vi "UI_(02B)_Switch_to_offline_mode.vi"(6 "error in (no error)":errorcluster, 9 "Settings cluster in":T1={"Defaults"={"Default User"=0.0, "VISA Resource Name "="", "Histogram parameters"={"max"=300.0, "min"=0.0, "# bins"=10, "threshold"=8.0, "thr. type"=enum."higher accepted"}}, "Recording and saving"={"Researcher name"="", "Name prefix"="", "Data post-processing"={"Filter type"=enum."Savitzky-Golay", "Length"=31, "Order"=3}, "Stop at"=0.0, "\"Stop at\" enabled"=FALSE, "Default save folder path"=path "", "Acquisition FPS"=enum."Max"}, "Geometry"={"Sensor board size"=enum."", "Bridge swap"=FALSE, "Twisted neck"=FALSE, "Bridge H. offset"=0.0, "Bridge V. offset"=0.0, "Magnets orientation"=0.0, "Cage type"=0, "Cage parameters"={"Round"=variant(i16 0), "Square"=variant(u16 0), "Donut-maze"=variant(u16 0), "T-maze"=variant(u8 0), "Sociability-maze"=variant(u8 0)}}, "IO parameters"={"IO general config."=0, "IO 1 configuration"=0, "IO 2 configuration"=0, "IO 3 configuration"=0, "IO 4 configuration"=0, "Activate ext. RS-232"=0, "IO inversion config."=0, "Sync capability"=1}, "Conditions presets array"=[{"Enabled"=FALSE, "Name"="", "Specifier(s)"=[], "Response"={"Response type"=enum."Air puff", "TTL port"=enum."Port 1", "TTL pulse length, ms"=0.0}, "Has been set"=FALSE}, {"Enabled"=FALSE, "Name"="", "Specifier(s)"=[], "Response"={"Response type"=enum."Air puff", "TTL port"=enum."Port 1", "TTL pulse length, ms"=0.0}, "Has been set"=FALSE}, {"Enabled"=FALSE, "Name"="", "Specifier(s)"=[], "Response"={"Response type"=enum."Air puff", "TTL port"=enum."Port 1", "TTL pulse length, ms"=0.0}, "Has been set"=FALSE}, {"Enabled"=FALSE, "Name"="", "Specifier(s)"=[], "Response"={"Response type"=enum."Air puff", "TTL port"=enum."Port 1", "TTL pulse length, ms"=0.0}, "Has been set"=FALSE}, {"Enabled"=FALSE, "Name"="", "Specifier(s)"=[], "Response"={"Response type"=enum."Air puff", "TTL port"=enum."Port 1", "TTL pulse length, ms"=0.0}, "Has been set"=FALSE}, {"Enabled"=FALSE, "Name"="", "Specifier(s)"=[], "Response"={"Response type"=enum."Air puff", "TTL port"=enum."Port 1", "TTL pulse length, ms"=0.0}, "Has been set"=FALSE}, {"Enabled"=FALSE, "Name"="", "Specifier(s)"=[], "Response"={"Response type"=enum."Air puff", "TTL port"=enum."Port 1", "TTL pulse length, ms"=0.0}, "Has been set"=FALSE}, {"Enabled"=FALSE, "Name"="", "Specifier(s)"=[], "Response"={"Response type"=enum."Air puff", "TTL port"=enum."Port 1", "TTL pulse length, ms"=0.0}, "Has been set"=FALSE}, {"Enabled"=FALSE, "Name"="", "Specifier(s)"=[], "Response"={"Response type"=enum."Air puff", "TTL port"=enum."Port 1", "TTL pulse length, ms"=0.0}, "Has been set"=FALSE}, {"Enabled"=FALSE, "Name"="", "Specifier(s)"=[], "Response"={"Response type"=enum."Air puff", "TTL port"=enum."Port 1", "TTL pulse length, ms"=0.0}, "Has been set"=FALSE}, {"Enabled"=FALSE, "Name"="", "Specifier(s)"=[], "Response"={"Response type"=enum."Air puff", "TTL port"=enum."Port 1", "TTL pulse length, ms"=0.0}, "Has been set"=FALSE}, {"Enabled"=FALSE, "Name"="", "Specifier(s)"=[], "Response"={"Response type"=enum."Air puff", "TTL port"=enum."Port 1", "TTL pulse length, ms"=0.0}, "Has been set"=FALSE}, {"Enabled"=FALSE, "Name"="", "Specifier(s)"=[], "Response"={"Response type"=enum."Air puff", "TTL port"=enum."Port 1", "TTL pulse length, ms"=0.0}, "Has been set"=FALSE}, {"Enabled"=FALSE, "Name"="", "Specifier(s)"=[], "Response"={"Response type"=enum."Air puff", "TTL port"=enum."Port 1", "TTL pulse length, ms"=0.0}, "Has been set"=FALSE}], "Calibration parameters"={"Timing calibration sw/hw"=1.0, "True FPS"=80.0, "True frame time, s"=0.0125, "Disp. calibration info"=[]}, "Settings loaded OK"=FALSE} {"Calibration parameters"."True frame time, s" format="%.10g"; "Calibration parameters"."Disp. calibration info"."Speed, µl per ms" format="%.3g"; "Calibration parameters"."True FPS" format="%.10g"; "Calibration parameters"."Timing calibration sw/hw" format="%.10g"; "Conditions presets array"."Specifier(s)"."Validity criteria(s)"."Validity value" min=0.0 step=0.1 format="%.2g"; "Conditions presets array"."Specifier(s)"."Value" step=1.0 format="%#.2g"; "Recording and saving"."Data post-processing"."Order" min=3 max=11 step=2; "Recording and saving"."Data post-processing"."Length" min=5 max=301 step=2; "Geometry"."Cage type" items=["Round", "Square", "Donut-maze", "T-maze", "Sociability maze", ""]}, 10 "All references in":T21) -> (0 "error out":errorcluster, 2 "Settings cluster out":T1={"Defaults"={"Default User"=0.0, "VISA Resource Name "="", "Histogram parameters"={"max"=300.0, "min"=0.0, "# bins"=10, "threshold"=8.0, "thr. type"=enum."higher accepted"}}, "Recording and saving"={"Researcher name"="", "Name prefix"="", "Data post-processing"={"Filter type"=enum."Savitzky-Golay", "Length"=31, "Order"=3}, "Stop at"=0.0, "\"Stop at\" enabled"=FALSE, "Default save folder path"=path "", "Acquisition FPS"=enum."Max"}, "Geometry"={"Sensor board size"=enum."", "Bridge swap"=FALSE, "Twisted neck"=FALSE, "Bridge H. offset"=0.0, "Bridge V. offset"=0.0, "Magnets orientation"=0.0, "Cage type"=0, "Cage parameters"={"Round"=variant(i16 0), "Square"=variant(u16 0), "Donut-maze"=variant(u16 0), "T-maze"=variant(u8 0), "Sociability-maze"=variant(u8 0)}}, "IO parameters"={"IO general config."=0, "IO 1 configuration"=0, "IO 2 configuration"=0, "IO 3 configuration"=0, "IO 4 configuration"=0, "Activate ext. RS-232"=0, "IO inversion config."=0, "Sync capability"=1}, "Conditions presets array"=[{"Enabled"=FALSE, "Name"="", "Specifier(s)"=[], "Response"={"Response type"=enum."Air puff", "TTL port"=enum."Port 1", "TTL pulse length, ms"=0.0}, "Has been set"=FALSE}, {"Enabled"=FALSE, "Name"="", "Specifier(s)"=[], "Response"={"Response type"=enum."Air puff", "TTL port"=enum."Port 1", "TTL pulse length, ms"=0.0}, "Has been set"=FALSE}, {"Enabled"=FALSE, "Name"="", "Specifier(s)"=[], "Response"={"Response type"=enum."Air puff", "TTL port"=enum."Port 1", "TTL pulse length, ms"=0.0}, "Has been set"=FALSE}, {"Enabled"=FALSE, "Name"="", "Specifier(s)"=[], "Response"={"Response type"=enum."Air puff", "TTL port"=enum."Port 1", "TTL pulse length, ms"=0.0}, "Has been set"=FALSE}, {"Enabled"=FALSE, "Name"="", "Specifier(s)"=[], "Response"={"Response type"=enum."Air puff", "TTL port"=enum."Port 1", "TTL pulse length, ms"=0.0}, "Has been set"=FALSE}, {"Enabled"=FALSE, "Name"="", "Specifier(s)"=[], "Response"={"Response type"=enum."Air puff", "TTL port"=enum."Port 1", "TTL pulse length, ms"=0.0}, "Has been set"=FALSE}, {"Enabled"=FALSE, "Name"="", "Specifier(s)"=[], "Response"={"Response type"=enum."Air puff", "TTL port"=enum."Port 1", "TTL pulse length, ms"=0.0}, "Has been set"=FALSE}, {"Enabled"=FALSE, "Name"="", "Specifier(s)"=[], "Response"={"Response type"=enum."Air puff", "TTL port"=enum."Port 1", "TTL pulse length, ms"=0.0}, "Has been set"=FALSE}, {"Enabled"=FALSE, "Name"="", "Specifier(s)"=[], "Response"={"Response type"=enum."Air puff", "TTL port"=enum."Port 1", "TTL pulse length, ms"=0.0}, "Has been set"=FALSE}, {"Enabled"=FALSE, "Name"="", "Specifier(s)"=[], "Response"={"Response type"=enum."Air puff", "TTL port"=enum."Port 1", "TTL pulse length, ms"=0.0}, "Has been set"=FALSE}, {"Enabled"=FALSE, "Name"="", "Specifier(s)"=[], "Response"={"Response type"=enum."Air puff", "TTL port"=enum."Port 1", "TTL pulse length, ms"=0.0}, "Has been set"=FALSE}, {"Enabled"=FALSE, "Name"="", "Specifier(s)"=[], "Response"={"Response type"=enum."Air puff", "TTL port"=enum."Port 1", "TTL pulse length, ms"=0.0}, "Has been set"=FALSE}, {"Enabled"=FALSE, "Name"="", "Specifier(s)"=[], "Response"={"Response type"=enum."Air puff", "TTL port"=enum."Port 1", "TTL pulse length, ms"=0.0}, "Has been set"=FALSE}, {"Enabled"=FALSE, "Name"="", "Specifier(s)"=[], "Response"={"Response type"=enum."Air puff", "TTL port"=enum."Port 1", "TTL pulse length, ms"=0.0}, "Has been set"=FALSE}], "Calibration parameters"={"Timing calibration sw/hw"=1.0, "True FPS"=80.0, "True frame time, s"=0.0125, "Disp. calibration info"=[]}, "Settings loaded OK"=FALSE} {"Calibration parameters"."True frame time, s" format="%.10g"; "Calibration parameters"."Disp. calibration info"."Speed, µl per ms" format="%.3g"; "Calibration parameters"."True FPS" format="%.10g"; "Calibration parameters"."Timing calibration sw/hw" format="%.10g"; "Conditions presets array"."Specifier(s)"."Validity criteria(s)"."Validity value" min=0.0 step=0.1 format="%.2g"; "Conditions presets array"."Specifier(s)"."Value" step=1.0 format="%#.2g"; "Recording and saving"."Data post-processing"."Order" min=3 max=11 step=2; "Recording and saving"."Data post-processing"."Length" min=5 max=301 step=2; "Geometry"."Cage type" items=["Round", "Square", "Donut-maze", "T-maze", "Sociability maze", ""]}, 3 "All references out":T21)   [LabVIEW 2018, in "Tracker.lvlib"]
uses:
  Tracker.lvlib
  Controls/CTL_All_References.ctl
  Controls/CTL_Controls_References.ctl
  Controls/CTL_Indicators_References.ctl
  Common/Typedefs/CTL_Panes_and_VIs_References.ctl
  Controls/CTL_Histogram_Properties.ctl
  <vilib>/Utility/miscctls.llb/LVRangeTypeDef.ctl
  Controls/CTL_Settings_cluster.ctl
  Controls/CTL_Histogram_parameters.ctl
  Controls/CTL_Filter_selector.ctl
  Controls/CTL_Acquisition_speed_selector.ctl
  Common/Typedefs/CTL_Segmented_plot_parameters_2.ctl
  Libraries/Cage Diagram/Typedefs/CTL_Cage_type.ctl
  Controls/CTL_Cage_all_segmentation_params_set.ctl
  Controls/CTL_IO_params_cluster.ctl
  Controls/CTL_Conditions_Array.ctl
  Controls/CTL_Conditions_Cluster.ctl
  Controls/CTL_Condition_type.ctl
  Controls/CTL_Comparison_type.ctl
  Controls/CTL_Validity_check_criteria.ctl
  Controls/CTL_Response_info.ctl
  Controls/CTL_Condition_response_type.ctl
  Controls/CTL_Reponse_port_info.ctl
  Controls/CTL_Calibration_parameters.ctl
  Controls/CTL_Dispenser_calibration_info.ctl
  <vilib>/Utility/error.llb/Error Cluster From Error Code.vi
  <vilib>/ErrorRing/Error Ring.xnode
  Common_Resources.lvlib
  Libraries/Cage Diagram/Cage Diagram.lvlib
panel:
  in  "Histogram initialization cluster":T19={"X Scale.Range"={"Minimum"=0.0, "Maximum"=13.0, "Increment"=1.0, "Minor Increment"=1.0, "Start"=0.0}, "Caption.Text"="Zone preference (normalized)", "X Scale.Offset and Multiplier:Multiplier"=1.0, "X Scale.Offset and Multiplier:Offset"=0.0, "X Scale.Scale Fit"=2, "X Scale.Display Format:Precision"=0, "Y Scale.Mapping Mode"=0, "Zones preference empty initialized array"=[0, 0, 0, 0, 0, 0, 0, 0, 0, 0, 0, 0, 0, 0], "Plot.Fill/Point Color"=15790320}
  out "Panes references":T24
  out "Controls references params":string[][](array[string])
  out "Indicators references params":string[][](array[string])
  out "Indicators references":T23
  out "Controls references":T22
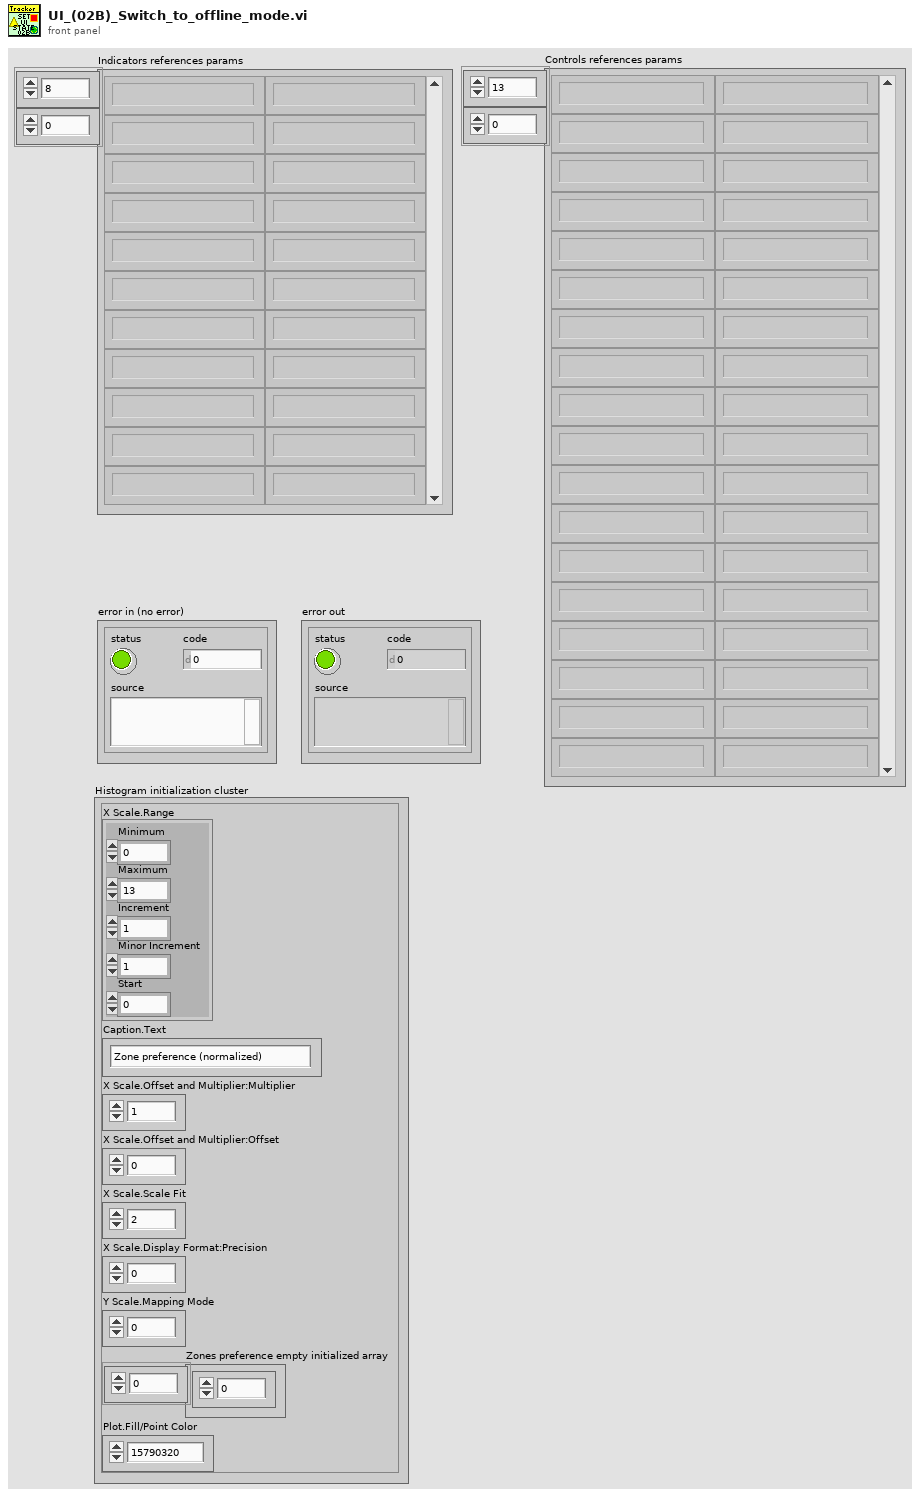
[diagram p1: front panel]
types:
  T1 = typedef "Common_Resources.lvlib/CTL_Settings_cluster.ctl" = cluster{"Defaults":cluster{"Default User":dbl, "VISA Resource Name ":string, "Histogram parameters":T2}, "Recording and saving":cluster{"Researcher name":string, "Name prefix":string, "Data post-processing":T3, "Stop at":dbl, "\"Stop at\" enabled":bool, "Default save folder path":path, "Acquisition FPS":T4}, "Geometry":T5, "IO parameters":T8, "Conditions presets array":T9, "Calibration parameters":T17, "Settings loaded OK":bool}
  T2 = typedef "Common_Resources.lvlib/CTL_Histogram_parameters.ctl" = cluster{"max":dbl, "min":dbl, "# bins":i32, "threshold":dbl, "thr. type":enum16{"higher accepted", "lower accepted"}}
  T3 = typedef "Common_Resources.lvlib/CTL_Filter_selector.ctl" = cluster{"Filter type":enum16{"None", "Savitzky-Golay"}, "Length":i32, "Order":i32}
  T4 = typedef "Common_Resources.lvlib/CTL_Acquisition_speed_selector.ctl" = enum16{"Max", "Optimal", "Eco"}
  T5 = typedef "Common_Resources.lvlib/CTL_Segmented_plot_parameters_2.ctl" = cluster{"Sensor board size":enum16{"", "Large"}, "Bridge swap":bool, "Twisted neck":bool, "Bridge H. offset":sgl, "Bridge V. offset":sgl, "Magnets orientation":sgl, "Cage type":T6, "Cage parameters":T7}
  T6 = typedef "Cage Diagram.lvlib/CTL_Cage_type.ctl" = u16
  T7 = typedef "Common_Resources.lvlib/CTL_Cage_all_segmentation_params_set.ctl" = cluster{"Round":variant, "Square":variant, "Donut-maze":variant, "T-maze":variant, "Sociability-maze":variant}
  T8 = typedef "Common_Resources.lvlib/CTL_IO_params_cluster.ctl" = cluster{"IO general config.":u16, "IO 1 configuration":u16, "IO 2 configuration":u16, "IO 3 configuration":u16, "IO 4 configuration":u16, "Activate ext. RS-232":u16, "IO inversion config.":u16, "Sync capability":u8}
  T9 = typedef "Common_Resources.lvlib/CTL_Conditions_Array.ctl" = T10[]
  T10 = typedef "Common_Resources.lvlib/CTL_Conditions_Cluster.ctl" = cluster{"Enabled":bool, "Name":string, "Specifier(s)":cluster{"Specifier enabled":bool, "Condition type":T11, "Comparison type":T12, "Value":dbl, "Validity criteria(s)":cluster{"V. check enabled":bool, "Criteria":T13, "Validity value":dbl}[]}[], "Response":T14, "Has been set":bool}
  T11 = typedef "Common_Resources.lvlib/CTL_Condition_type.ctl" = enum16{"Speed", "Zone", "Angle to wall"}
  T12 = typedef "Common_Resources.lvlib/CTL_Comparison_type.ctl" = enum16{"Less", "Less or Equal", "Equal", "Greater or Equal", "Greater", "Not Equal"}
  T13 = typedef "Common_Resources.lvlib/CTL_Validity_check_criteria.ctl" = enum16{"Running bout (seconds)", "Running bout (meters)"}
  T14 = typedef "Common_Resources.lvlib/CTL_Response_info.ctl" = cluster{"Response type":T15, "TTL port":T16, "TTL pulse length, ms":dbl}
  T15 = typedef "Common_Resources.lvlib/CTL_Condition_response_type.ctl" = enum16{"None", "Air puff", "Liquid reward", "TTL pulse", "TTL pulse (ubr)", "TTL signal"}
  T16 = typedef "Common_Resources.lvlib/CTL_Reponse_port_info.ctl" = enum16{"Port 1", "Port 2", "Port 3", "Port 4"}
  T17 = typedef "Common_Resources.lvlib/CTL_Calibration_parameters.ctl" = cluster{"Timing calibration sw/hw":dbl, "True FPS":dbl, "True frame time, s":dbl, "Disp. calibration info":T18}
  T18 = typedef "Common_Resources.lvlib/CTL_Dispenser_calibration_info.ctl" = cluster{"Channel":u8, "Speed, µl per ms":dbl}[]
  T19 = typedef "Common_Resources.lvlib/CTL_Histogram_Properties.ctl" = cluster{"X Scale.Range":T20, "Caption.Text":string, "X Scale.Offset and Multiplier:Multiplier":dbl, "X Scale.Offset and Multiplier:Offset":dbl, "X Scale.Scale Fit":u8, "X Scale.Display Format:Precision":u8, "Y Scale.Mapping Mode":u8, "Zones preference empty initialized array":i32[], "Plot.Fill/Point Color":u32}
  T20 = typedef "LVRangeTypeDef.ctl" = cluster{"Minimum":dbl, "Maximum":dbl, "Increment":dbl, "Minor Increment":dbl, "Start":dbl}
  T21 = typedef "Common_Resources.lvlib/CTL_All_References.ctl" = cluster{"Controls references":T22, "Indicators references":T23, "Service references":T24}
  T22 = typedef "Common_Resources.lvlib/CTL_Controls_References.ctl" = cluster{"Check HW connection":refnum<vi>, "Save settings":refnum<vi>, "Reset zones":refnum<vi>, "Reset stimuli":refnum<vi>, "Record/Stop":refnum<vi>, "Reset barplot":refnum<vi>, "Multiplyer of chart RX":refnum<vi>, "Show zones":refnum<vi>, "Show magnets":refnum<vi>, "Show heatmap":refnum<vi>, "Show full track":refnum<vi>, "Open File":refnum<vi>, "Play/Pause":refnum<vi>, "Trace, s":refnum<vi>, "Playback speed":refnum<vi>, "Timeline":refnum<vi>, "By Zone stim. setup":refnum<vi>, "Set/Rec and Analyse Tab":refnum<vi>, "Cage radial segmentation":refnum<vi>, "Set IO config":refnum<vi>, "Rainbow (time)":refnum<vi>, "Rainbow (speed)":refnum<vi>, "Add Reward":refnum<vi>, "Modify Reward":refnum<vi>, "Delete Reward":refnum<vi>, "Speed threshold, mm/s":refnum<vi>, "Start Over":refnum<vi>}
  T23 = typedef "Common_Resources.lvlib/CTL_Indicators_References.ctl" = cluster{"HW info":refnum<vi>, "Port":refnum<vi>, "Ready":refnum<vi>, "IO status indicator":refnum<vi>, "Current Time":refnum<vi>, "Record timestamp":refnum<vi>, "Mouse speed":refnum<vi>, "Mouse speed, mm/s":refnum<vi>, "Running, perc. of time":refnum<vi>, "Histograms":refnum<vi>, "Cage size":refnum<vi>, "Reward":refnum<vi>, "Current zone":refnum<vi>, "Run length, m":refnum<vi>}
  T24 = typedef "Common_Resources.lvlib/CTL_Panes_and_VIs_References.ctl" = cluster{"Pane":refnum<vi>, "This VI":refnum<vi>, "Menu":refnum<k9>}
  T25 = enum8{"Enabled", "Disabled", "Disabled and Grayed Out"}
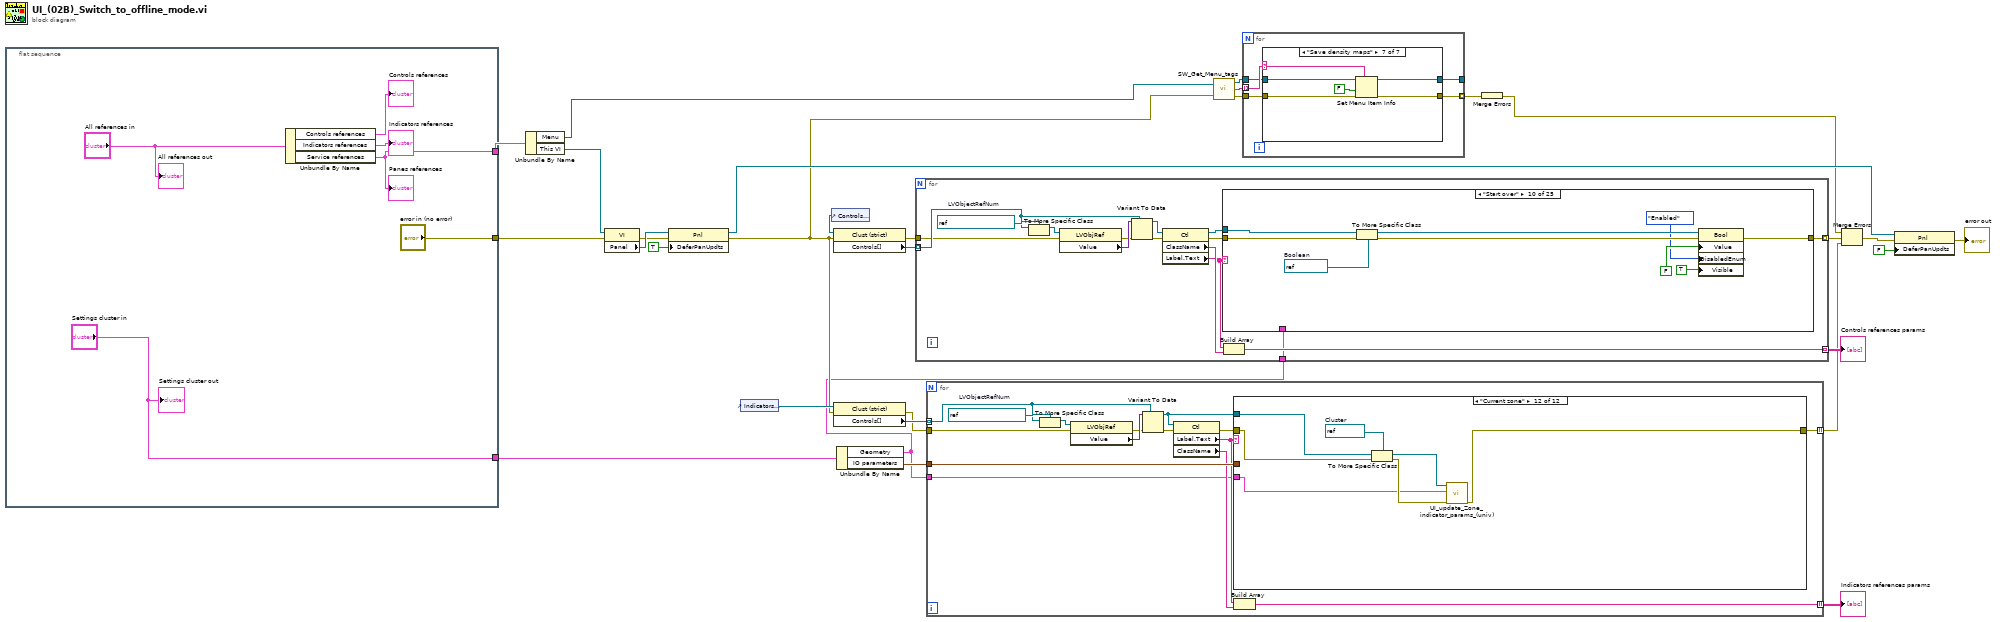
[diagram p0: block diagram]
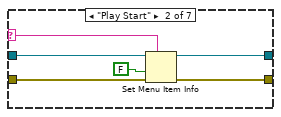
[diagram p3: hidden frame]
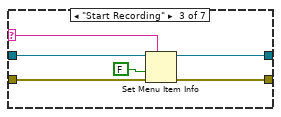
[diagram p4: hidden frame]
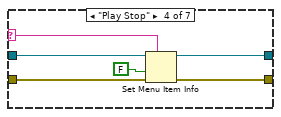
[diagram p5: hidden frame]
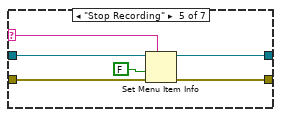
[diagram p6: hidden frame]
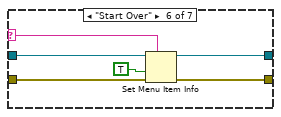
[diagram p7: hidden frame]
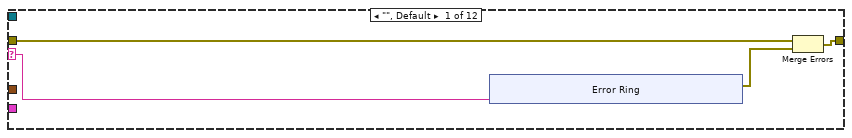
[diagram p8: hidden frame]
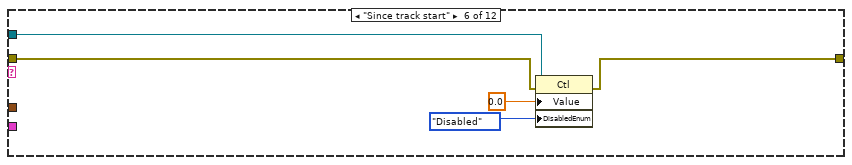
[diagram p13: hidden frame]
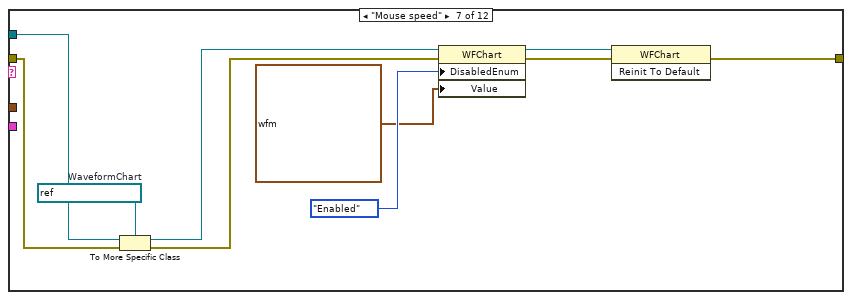
[diagram p14: hidden frame]
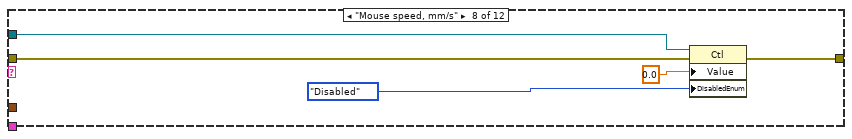
[diagram p15: hidden frame]
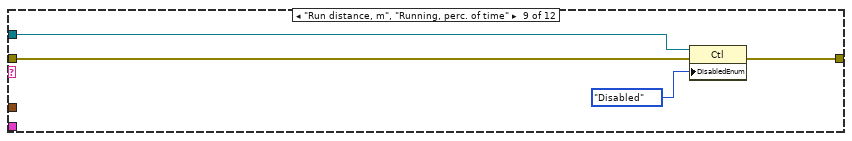
[diagram p16: hidden frame]
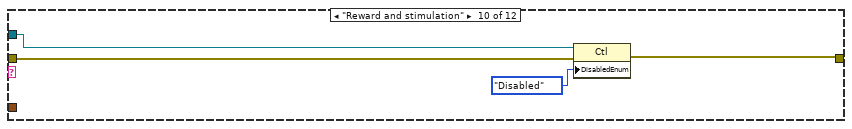
[diagram p17: hidden frame]
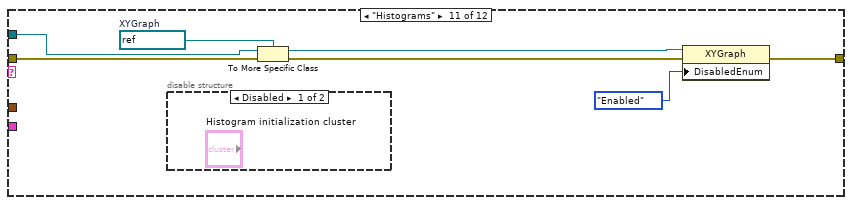
[diagram p18: hidden frame]
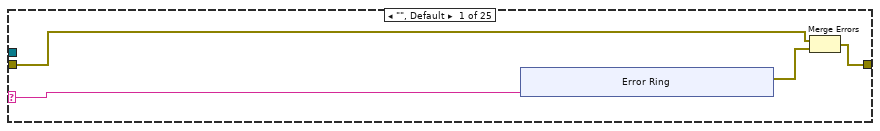
[diagram p20: hidden frame]
diagram:
  n1 = flat-sequence {
    tunnel: [w33] -> w24
    tunnel: ["Settings cluster in"] -> w11
    tunnel: ["error in (no error)"] -> w9
    frame #0 {
      n2 = Unbundle By Name("All references in") -> ("Controls references"=→"Controls references":T22, "Indicators references"=→"Indicators references":T23, "Service references"=w33:T24)
      "Panes references" <- w33
      "All references out" <- "All references in"
      "Settings cluster out" <- "Settings cluster in"
    }
  }
  n3 = Unbundle By Name(w24) -> ("Menu"=w4:refnum<k9>, "This VI"=w21:refnum<vi>)
  n4 = property class="VI"(reference=w21, error in=w9) -> (error out=w14:errorcluster, "Panel"=w23:refnum<vi>)  [unwired: 1 out]
  n5 = property class="Pnl"(reference=w23, error in=w14, "DeferPanUpdts"=TRUE ("Defer Panel Updates")) -> (reference out=w15:refnum<vi>, error out=w3:errorcluster)
  n6 = control-ref of="Indicators references"() -> (w27:refnum<vi>)
  n7 = control-ref of="Controls references"() -> (w29:refnum<vi>)
  n8 = property class="Clust (strict)"(reference=w29, error in=w3) -> (error out=w20:errorcluster, "Controls[]"=w30:refnum<vi>[])  [unwired: 1 out]
  n9 = property class="Clust (strict)"(reference=w27, error in=w3) -> (error out=w19:errorcluster, "Controls[]"=w28:refnum<vi>[])  [unwired: 1 out]
  n10 = Unbundle By Name(w11) -> ("Geometry"=w1:T5, "IO parameters"=w10:T8)
  n11 = for {
    tunnel: w30 -> [w48] mode=indexing
    tunnel: [w45] -> w25 mode=indexing
    tunnel: w20 -> [w44]
    tunnel: [w40] -> w12 mode=indexing
    tunnel: w1 -> [w37]
    w50 = refnum<vi> refnum  # LVObjectRefNum
    n12 = To More Specific Class(target class=w50, reference=w48) -> (specific class reference=w51:refnum<vi>)  [unwired: 1 in, 1 out]
    n13 = property class="LVObjRef"(reference=w51, error in=w44) -> (error out=w43:errorcluster, "Value"=w49:variant)  [unwired: 1 out]
    n14 = Variant To Data(error in=w43, type=w48, Variant=w49) -> (data=w47:refnum<vi>, error out=w42:errorcluster)
    n15 = property class="Ctl"(reference=w47, error in=w42) -> (reference out=w38:refnum<vi>, error out=w39:errorcluster, "ClassName"=w46:string, "Label.Text"=w41:string)
    n16 = case shown="\"Start over\"" w41 {
      selector: w41 -> [w52 _ _ _ _ _ _ _ _ _ _ _ _ _ _ _ _ _ _ _ _ _ _ _ _]
      tunnel: [w54 w64 w70 w77 w78 w79 w80 w81 w85 w94 w102 w110 w118 w124 w132 w140 w146 w152 w162 w168 w171 w178 w186 w193 w199] -> w40
      tunnel: w39 -> [w55 w65 w75 w77 w78 w79 w80 w81 w87 w96 w104 w112 w120 w125 w134 w141 w148 w153 w165 w168 w173 w180 w188 w195 w199]
      tunnel: w38 -> [_ w63 w76 _ _ _ _ _ w90 w99 w107 w115 w123 w126 w133 w139 w151 w159 w166 _ w176 w183 w191 w198 _]
      tunnel: w37 -> [_ _ _ _ _ _ _ _ _ _ _ _ _ _ _ _ _ _ _ _ _ _ _ _ _]
      frame "", Default {
        n17 = xnode "Error Ring"("parameter 0"=w52) -> ("error out"=w53:errorcluster)
        n18 = Merge Errors(w55, w53) -> (w54:errorcluster)
      }
      frame "Cage radial segmentation" {
        w66 = refnum<vi> refnum  # Cluster
        n19 = To More Specific Class(target class=w66, reference=w63, error in=w65) -> (specific class reference=w67:refnum<vi>, error out=w68:errorcluster)
        n20 = property class="Clust"(reference=w67, error in=w68, "DisabledEnum"=T25."Disabled and Grayed Out" ("Disabled")) -> (error out=w64:errorcluster)  [unwired: 1 out]
      }
      frame "Set/Rec and Analyse Tab" {
        w74 = refnum<vi> refnum  # TabControl
        n21 = To More Specific Class(target class=w74, reference=w76, error in=w75) -> (specific class reference=w72:refnum<vi>, error out=w73:errorcluster)
        n22 = property class="TabCtl"(reference=w72, error in=w73, "Value"=enum32{"Settings", "Recording and Analysis"}."Recording and Analysis" ("Set/Rec and Analyse Tab")) -> (error out=w70:errorcluster)  [unwired: 1 out]
      }
      frame "Check HW connection" {
      }
      frame "Save settings" {
      }
      frame "Set IO config" {
      }
      frame "Reset zones" {
      }
      frame "Reset stimuli" {
      }
      frame "Record/Stop" {
        w89 = refnum<vi> refnum  # Boolean
        n23 = To More Specific Class(target class=w89, reference=w90, error in=w87) -> (specific class reference=w88:refnum<vi>, error out=w86:errorcluster)
        n24 = property class="Bool"(reference=w88, error in=w86, "Value"=FALSE, "DisabledEnum"=T25."Disabled and Grayed Out" ("Disabled"), "Visible"=FALSE) -> (error out=w85:errorcluster)  [unwired: 1 out]
      }
      frame "Start over" {
        w98 = refnum<vi> refnum  # Boolean
        n25 = To More Specific Class(target class=w98, reference=w99, error in=w96) -> (specific class reference=w97:refnum<vi>, error out=w95:errorcluster)
        n26 = property class="Bool"(reference=w97, error in=w95, "Value"=FALSE, "DisabledEnum"=T25."Enabled" ("Disabled"), "Visible"=TRUE) -> (error out=w94:errorcluster)  [unwired: 1 out]
      }
      frame "Reset barplot" {
        w106 = refnum<vi> refnum  # Boolean
        n27 = To More Specific Class(target class=w106, reference=w107, error in=w104) -> (specific class reference=w105:refnum<vi>, error out=w103:errorcluster)
        n28 = property class="Bool"(reference=w105, error in=w103, "Value"=FALSE, "DisabledEnum"=T25."Enabled" ("Disabled")) -> (error out=w102:errorcluster)  [unwired: 1 out]
      }
      frame "Multiplyer of chart RX" {
        w114 = refnum<vi> refnum  # Slide
        n29 = To More Specific Class(target class=w114, reference=w115, error in=w112) -> (specific class reference=w113:refnum<vi>, error out=w111:errorcluster)
        n30 = property class="Slide"(reference=w113, error in=w111, "Value"=u8 1, "DisabledEnum"=T25."Enabled" ("Disabled")) -> (error out=w110:errorcluster)  [unwired: 1 out]
      }
      frame "Show zones" {
        w122 = refnum<vi> refnum  # Boolean
        n31 = To More Specific Class(target class=w122, reference=w123, error in=w120) -> (specific class reference=w121:refnum<vi>, error out=w119:errorcluster)
        n32 = property class="Bool"(reference=w121, error in=w119, "Val(Sgnl)"=FALSE, "DisabledEnum"=T25."Enabled" ("Disabled")) -> (error out=w118:errorcluster)  [unwired: 1 out]
      }
      frame "Show magnets" {
        w127 = refnum<vi> refnum  # Boolean
        n33 = To More Specific Class(target class=w127, reference=w126, error in=w125) -> (specific class reference=w131:refnum<vi>, error out=w130:errorcluster)
        n34 = property class="Bool"(reference=w131, error in=w130, "Val(Sgnl)"=FALSE, "DisabledEnum"=T25."Enabled" ("Disabled")) -> (error out=w124:errorcluster)  [unwired: 1 out]
      }
      frame "Rainbow (speed)", "Rainbow (time)" {
        w135 = refnum<vi> refnum  # Boolean
        n35 = To More Specific Class(target class=w135, reference=w133, error in=w134) -> (specific class reference=w137:refnum<vi>, error out=w138:errorcluster)
        n36 = property class="Bool"(reference=w137, error in=w138, "DisabledEnum"=T25."Enabled" ("Disabled")) -> (error out=w132:errorcluster)  [unwired: 1 out]
      }
      frame "Add Reward", "Modify Reward", "Remove Reward" {
        n37 = property class="Ctl"(reference=w139, error in=w141, "Value"=FALSE, "DisabledEnum"=T25."Disabled and Grayed Out" ("Disabled")) -> (error out=w140:errorcluster)  [unwired: 1 out]
      }
      frame "Show heatmap" {
        w150 = refnum<vi> refnum  # Boolean
        n38 = To More Specific Class(target class=w150, reference=w151, error in=w148) -> (specific class reference=w149:refnum<vi>, error out=w147:errorcluster)
        n39 = property class="Bool"(reference=w149, error in=w147, "Value"=FALSE, "DisabledEnum"=T25."Disabled and Grayed Out" ("Disabled")) -> (error out=w146:errorcluster)  [unwired: 1 out]
      }
      frame "Show full track" {
        w158 = refnum<vi> refnum  # Boolean
        n40 = To More Specific Class(target class=w158, reference=w159, error in=w153) -> (specific class reference=w157:refnum<vi>, error out=w156:errorcluster)
        n41 = property class="Bool"(reference=w157, error in=w156, "Val(Sgnl)"=TRUE, "DisabledEnum"=T25."Enabled" ("Disabled")) -> (error out=w152:errorcluster)  [unwired: 1 out]
      }
      frame "Open File" {
        w167 = refnum<vi> refnum  # Boolean
        n42 = To More Specific Class(target class=w167, reference=w166, error in=w165) -> (specific class reference=w164:refnum<vi>, error out=w163:errorcluster)
        n43 = property class="Bool"(reference=w164, error in=w163, "DisabledEnum"=T25."Enabled" ("Disabled"), "Value"=FALSE) -> (error out=w162:errorcluster)  [unwired: 1 out]
      }
      frame "Play/Pause" {
      }
      frame "Trace, s" {
        w175 = refnum<vi> refnum  # Slide
        n44 = To More Specific Class(target class=w175, reference=w176, error in=w173) -> (specific class reference=w174:refnum<vi>, error out=w172:errorcluster)
        n45 = property class="Slide"(reference=w174, error in=w172, "Value"=u8 5, "DisabledEnum"=T25."Enabled" ("Disabled")) -> (error out=w171:errorcluster)  [unwired: 1 out]
      }
      frame "Speed threshold" {
        w182 = refnum<vi> refnum  # Digital
        n46 = To More Specific Class(target class=w182, reference=w183, error in=w180) -> (specific class reference=w181:refnum<vi>, error out=w179:errorcluster)
        n47 = property class="DigNum"(reference=w181, error in=w179, "DisabledEnum"=T25."Enabled" ("Disabled")) -> (error out=w178:errorcluster)  [unwired: 1 out]
      }
      frame "Playback speed" {
        w190 = refnum<vi> refnum  # Ring
        n48 = To More Specific Class(target class=w190, reference=w191, error in=w188) -> (specific class reference=w189:refnum<vi>, error out=w187:errorcluster)
        n49 = property class="Ring"(reference=w189, error in=w187, "Value"=u8 120, "DisabledEnum"=T25."Enabled" ("Disabled")) -> (error out=w186:errorcluster)  [unwired: 1 out]
      }
      frame "Timeline" {
        w197 = refnum<vi> refnum  # Slide
        n50 = To More Specific Class(target class=w197, reference=w198, error in=w195) -> (specific class reference=w196:refnum<vi>, error out=w194:errorcluster)
        n51 = property class="Slide"(reference=w196, error in=w194, "DisabledEnum"=T25."Disabled and Grayed Out" ("Disabled")) -> (error out=w193:errorcluster)  [unwired: 1 out]
      }
      frame "By Zone stim. setup" {
      }
    }
    n52 = Build Array(w41, w46) -> (w45:string[])
  }
  "Controls references params" <- w25
  n53 = for {
    tunnel: w28 -> [w211] mode=indexing
    tunnel: [w201] -> w26 mode=indexing
    tunnel: w19 -> [w209]
    tunnel: [w205] -> w18 mode=indexing
    tunnel: w10 -> [w204]
    tunnel: w1 -> [w200]
    w213 = refnum<vi> refnum  # LVObjectRefNum
    n54 = To More Specific Class(target class=w213, reference=w211) -> (specific class reference=w214:refnum<vi>)  [unwired: 1 in, 1 out]
    n55 = property class="LVObjRef"(reference=w214, error in=w209) -> (error out=w208:errorcluster, "Value"=w212:variant)  [unwired: 1 out]
    n56 = Variant To Data(error in=w208, type=w211, Variant=w212) -> (data=w210:refnum<vi>, error out=w207:errorcluster)
    n57 = property class="Ctl"(reference=w210, error in=w207) -> (error out=w206:errorcluster, "Label.Text"=w203:string, "ClassName"=w202:string)  [unwired: 1 out]
    n58 = case shown="\"Current zone\"" w203 {
      selector: w203 -> [w215 _ _ _ _ _ _ _ _ _ _ _]
      tunnel: w210 -> [_ _ _ _ _ w230 w244 w249 w253 w254 w264 w267]
      tunnel: w206 -> [w218 w226 w227 w228 w229 w232 w240 w248 w252 w256 w260 w268]
      tunnel: [w217 w226 w227 w228 w229 w231 w236 w247 w251 w255 w263 w266] -> w205
      tunnel: w204 -> [_ _ _ _ _ _ _ _ _ _ _ _]
      tunnel: w200 -> [_ _ _ _ _ _ _ _ _ _ _ w265]
      frame "", Default {
        n59 = xnode "Error Ring"("parameter 0"=w215) -> ("error out"=w216:errorcluster)
        n60 = Merge Errors(w218, w216) -> (w217:errorcluster)
      }
      frame "Cage size", "HW info", "Port" {
      }
      frame "Ready" {
      }
      frame "IO status indicator" {
      }
      frame "Current Time" {
      }
      frame "Since track start" {
        n61 = property class="Ctl"(reference=w230, error in=w232, "Value"=0.0, "DisabledEnum"=T25."Disabled" ("Disabled")) -> (error out=w231:errorcluster)  [unwired: 1 out]
      }
      frame "Mouse speed" {
        w241 = refnum<vi> refnum  # WaveformChart
        n62 = To More Specific Class(target class=w241, reference=w244, error in=w240) -> (specific class reference=w242:refnum<vi>, error out=w239:errorcluster)
        n63 = property class="WFChart"(reference=w242, error in=w239, "DisabledEnum"=T25."Enabled" ("Disabled"), "Value"=waveform(dbl)[] [{"t0"=timestamp(0 s since 1904-01-01), "dt"=1.0, "Y"=[0.0]}] ("History Data")) -> (reference out=w238:refnum<vi>, error out=w237:errorcluster)
        n64 = invoke class="WFChart" method="Reinit To Default"(reference=w238, error in=w237) -> (error out=w236:errorcluster)  [unwired: 1 in, 2 out]
      }
      frame "Mouse speed, mm/s" {
        n65 = property class="Ctl"(reference=w249, error in=w248, "Value"=0.0, "DisabledEnum"=T25."Disabled" ("Disabled")) -> (error out=w247:errorcluster)  [unwired: 1 out]
      }
      frame "Run distance, m", "Running, perc. of time" {
        n66 = property class="Ctl"(reference=w253, error in=w252, "DisabledEnum"=T25."Disabled" ("Disabled")) -> (error out=w251:errorcluster)  [unwired: 1 out]
      }
      frame "Reward and stimulation" {
        n67 = property class="Ctl"(reference=w254, error in=w256, "DisabledEnum"=T25."Disabled" ("Disabled")) -> (error out=w255:errorcluster)  [unwired: 1 out]
      }
      frame "Histograms" {
        w261 = refnum<vi> refnum  # XYGraph
        n68 = disable-structure shown="Disabled" {
          frame Disabled {
          }
          frame Enabled {
          }
        }
        n69 = To More Specific Class(target class=w261, reference=w264, error in=w260) -> (specific class reference=w262:refnum<vi>, error out=w259:errorcluster)
        n70 = property class="XYGraph"(reference=w262, error in=w259, "DisabledEnum"=T25."Enabled" ("Disabled")) -> (error out=w263:errorcluster)  [unwired: 1 out]
      }
      frame "Current zone" {
        w271 = refnum<vi> refnum  # Cluster
        n71 = To More Specific Class(target class=w271, reference=w267, error in=w268) -> (specific class reference=w269:refnum<vi>, error out=w270:errorcluster)
        n72 = call "UI_update_Zone_indicator_params_(univ).vi"("error in (no error)"=w270, "Geometry"=w265, "Zone indicator ref. in"=w269) -> ("error out"=w266:errorcluster)  [unwired: 7 in, 1 out]
      }
    }
    n73 = Build Array(w203, w202) -> (w201:string[])
  }
  "Indicators references params" <- w26
  n74 = call "SW_Get_Menu_tags.vi"("Menu ref in"=w4, "error in (no error)"=w3) -> ("Menu ref out"=w6:refnum<k9>, "(Sub)menu tags"=w8:string[], "error out"=w7:errorcluster)
  n75 = for {
    tunnel: w8 -> [w276] mode=indexing
    tunnel: w7 -> [w275]
    tunnel: [w274] -> w5 mode=indexing
    tunnel: [w273] -> _
    tunnel: w6 -> [w272]
    n76 = case shown="\"Save density maps\"" w276 {
      selector: w276 -> [_ w284 w290 w296 w302 w308 w314]
      tunnel: w275 -> [w278 w282 w288 w294 w300 w306 w312]
      tunnel: [w278 w281 w287 w293 w299 w305 w311] -> w274
      tunnel: [w277 w280 w286 w292 w298 w304 w310] -> w273
      tunnel: w272 -> [w277 w279 w285 w291 w297 w303 w309]
      frame "", Default {
      }
      frame "Play Start" {
        n77 = Set Menu Item Info(7:w284, 8:w282, 9:FALSE ("enabled"), 11:w279) -> (0:w281:errorcluster, 3:w280:refnum<k9>)  [unwired: 3 in]
      }
      frame "Start Recording" {
        n78 = Set Menu Item Info(7:w290, 8:w288, 9:FALSE ("enabled"), 11:w285) -> (0:w287:errorcluster, 3:w286:refnum<k9>)  [unwired: 3 in]
      }
      frame "Play Stop" {
        n79 = Set Menu Item Info(7:w296, 8:w294, 9:FALSE ("enabled"), 11:w291) -> (0:w293:errorcluster, 3:w292:refnum<k9>)  [unwired: 3 in]
      }
      frame "Stop Recording" {
        n80 = Set Menu Item Info(7:w302, 8:w300, 9:FALSE ("enabled"), 11:w297) -> (0:w299:errorcluster, 3:w298:refnum<k9>)  [unwired: 3 in]
      }
      frame "Start Over" {
        n81 = Set Menu Item Info(7:w308, 8:w306, 9:TRUE ("enabled"), 11:w303) -> (0:w305:errorcluster, 3:w304:refnum<k9>)  [unwired: 3 in]
      }
      frame "Save density maps" {
        n82 = Set Menu Item Info(7:w314, 8:w312, 9:FALSE ("enabled"), 11:w309) -> (0:w311:errorcluster, 3:w310:refnum<k9>)  [unwired: 3 in]
      }
    }
  }
  n83 = Merge Errors(w5) -> (w2:errorcluster)
  n84 = Merge Errors(w2, w12, w18) -> (w17:errorcluster)
  n85 = property class="Pnl"(reference=w15, error in=w17, "DeferPanUpdts"=FALSE ("Defer Panel Updates")) -> (error out=→"error out":errorcluster)  [unwired: 1 out]
